vi "Get Temp Filepath.vi"() -> (0 "Temp Settings Filepath":path)   [LabVIEW 2023, in "Error Manager.lvlib" / "Settings.lvclass"]
doc: "This VI generates a temporary, unique filename and filepath. A copy of the Error Manager settings file (ini file) will be saved with the new filename, at the new filepath. This copy will be deleted shortly after it is created.\n\nThe following implementation details help ensure that the path is unique:\n1. The temp filename contains the \"now\" UTC timestamp (ms accuracy)\n2. The temp filename contains a string of 12 random lowercase letters (serving as a GUID)\n\n<B>Example temp filename:</B> 2023-09-16 15-24-58.692 Error Manager Settings (comments removed) dokwnixxizdj.tmp\n<B>Example temp filepath (on Windows 11 computer):</B> C:\\Users\\<username>\\AppData\\Local\\Temp\\2023-09-16 15-24-58.692 Error Manager Settings (comments removed) dokwnixxizdj.tmp"
uses:
  Settings.lvclass
  <vilib>/Utility/sysdir.llb/System Directory Type.ctl
  ASCII Character Type (enum).ctl
  Generate Random ASCII Character.vi
  <vilib>/numeric/Random Number (Range).vi
  <vilib>/numeric/Random Number (Range) U64.vi
  <vilib>/numeric/sub_Random U32.vi
panel:
  out "Temp Filename":string
  out "Timestamp":string
  out "Temp Directory":path
  # "Development\nControls or indicators that are useful for development or testing, but which are not outputs of the VI."
  # "Input\nInputs to the VI"
  # "Output\nOutputs of the VI"
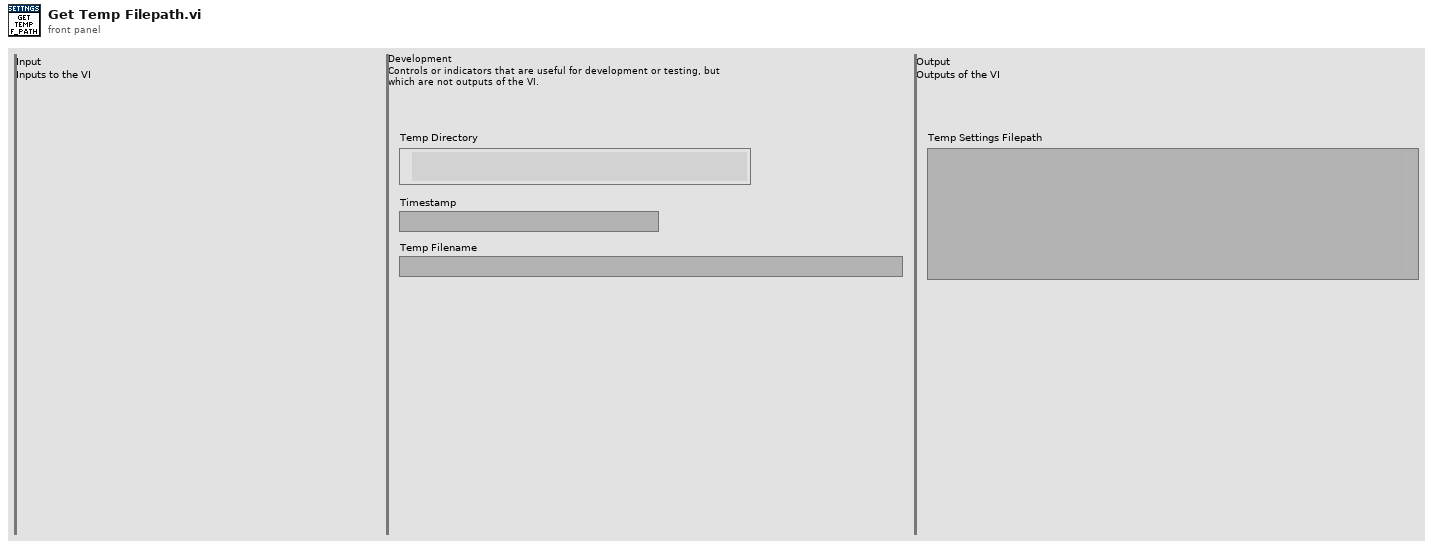
[diagram p1: front panel]
types:
  T1 = typedef "Error Manager.lvlib/Settings.lvclass/ASCII Character Type (enum).ctl" = enum16{"Lowercase Letter", "Uppercase Letter", "Digit", "Alphanumeric", "Printable Character", "Any ASCII Character [0x00 to 0xFF]"}
  T2 = typedef "System Directory Type.ctl" = i32
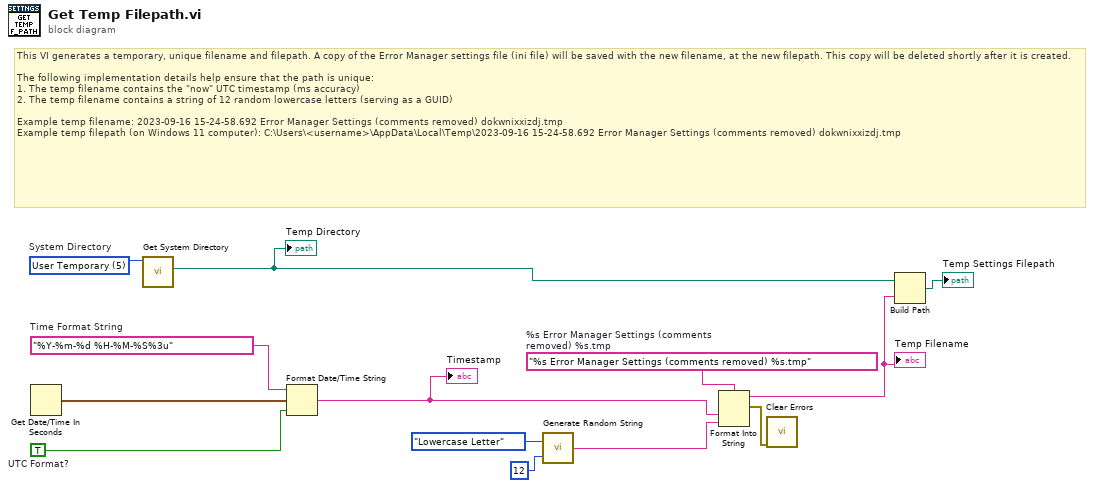
[diagram p0: block diagram]
diagram:
  w9 = "%s Error Manager Settings (comments removed) %s.tmp"  # %s Error Manager Settings (comments removed) %s.tmp
  w10 = "%Y-%m-%d %H-%M-%S%3u"  # Time Format String
  w11 = TRUE  # UTC Format?
  w13 = T2 5 items=["User Home"=0, "User Desktop"=1, "User Documents"=2, "User Application Data"=3, "User Preferences"=4, "User Temporary"=5, "Public Documents"=6, "Public Application Data"=7, "Public Preferences"=8, "Public Cache"=13, "System Core Libraries"=9, "System Installed Libraries"=10, "Application Files"=11, "Boot Volume Root"=12]  # System Directory
  # "This VI generates a temporary, unique filename and filepath. A copy of the Error Manager settings file (ini file) will be saved with the new filename, at the new filepath. This copy will be deleted shortly after it is created.\n\nThe following implementation details help ensure that the path is unique:\n1. The temp filename contains the \"now\" UTC timestamp (ms accuracy)\n2. The temp filename contains a string of 12 random lowercase letters (serving as a GUID)\n\nExample temp filename: 2023-09-16 15-24-58.692 Error Manager Settings (comments removed) dokwnixxizdj.tmp\nExample temp filepath (on Windows 11 computer): C:\\Users\\<username>\\AppData\\Local\\Temp\\2023-09-16 15-24-58.692 Error Manager Settings (comments removed) dokwnixxizdj.tmp"
  n1 = Get Date/Time In Seconds() -> (seconds since 1Jan1904=w12:timestamp)
  n2 = call <vilib>:"Get System Directory.vi"("system directory type"=w13) -> ("system directory"=w3:path)  [unwired: 10 in]
  "Temp Directory" <- w3
  n3 = Format Date/Time String(time format string (%c)=w10, seconds (now)=w12, UTC format=w11) -> (date/time string=w7:string)
  "Timestamp" <- w7
  n4 = call "Generate Random String.vi"("String Length (Default = 10)"=u32 12, "ASCII Character Type"=ASCII_Character_Type_(enum)."Lowercase Letter") -> ("Random String"=w8:string)
  n5 = Format Into String(format string=w9, w7, w8) -> (resulting string=w2:string, error out=w4:errorcluster)  [unwired: 2 in]
  "Temp Filename" <- w2
  n6 = call <vilib>:"Clear Errors.vi"("error in (no error)"=w4) -> ()  [unwired: 5 in, 2 out]
  n7 = Build Path(base path=w3, name or relative path=w2) -> (appended path=→"Temp Settings Filepath":path)
